vi "ELVIS III v1.0 Reset Encoder.vi"(8 "error in (no error)":errorcluster, 10 "Channel":T1, 11 "myRIO Ref In":T2) -> (0 "error out":errorcluster, 3 "myRIO Ref Out":T2)   [LabVIEW 2021]
uses:
  <vilib>/myRIO/Common/Instrument Driver Framework/Utilities/typedefs/myRIO v1.0 Reference.ctl
  <vilib>/myRIO/Common/Instrument Driver Framework/Utilities/typedefs/Generic FPGA Reference.ctl
  <vilib>/myRIO/Common/Instrument Driver Framework/myRIO v1.0/Encoder/typedefs/Encoder Channels Enum.ctl
  <vilib>/myRIO/Common/Instrument Driver Framework/ELVIS III v1.0/Encoder/typedefs/ELVIS III Encoder Channels FPGA Reference.ctl
  <vilib>/rvi/errors/niLvFpgaAdjustHostInterfaceError.vi
  <vilib>/rvi/interface/nirviReadWriteControl/nirviReadWriteControl.xnode
  <vilib>/rvi/interface/Simulation/niFpgaSimulationCallBeginRW.vi
  NiFpgaLv.dll
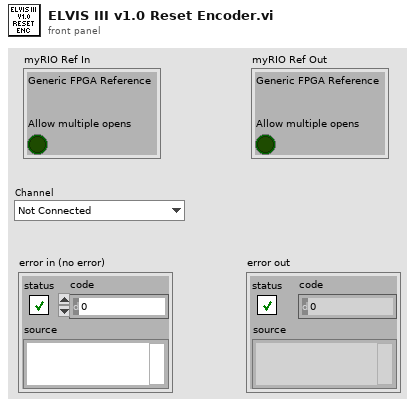
[diagram p1: front panel]
types:
  T1 = typedef "Encoder Channels Enum.ctl" = enum16{"Not Connected", "C/ENC0", "C/ENC1", "A/ENC", "A/ENC0", "A/ENC1", "A/ENC2", "A/ENC3", "A/ENC4", "A/ENC5", "A/ENC6", "A/ENC7", "A/ENC8", "A/ENC9", "B/ENC", "B/ENC0", "B/ENC1", "B/ENC2", "B/ENC3", "B/ENC4", "B/ENC5", "B/ENC6", "B/ENC7", "B/ENC8", "B/ENC9", "DIO/ENC0", "DIO/ENC1", "DIO/ENC2", "DIO/ENC3", "DIO/ENC4"}
  T2 = typedef "myRIO v1.0 Reference.ctl" = cluster{"Generic FPGA Reference":T3, "Allow multiple opens":bool}
  T3 = typedef "Generic FPGA Reference.ctl" = refnum<k20>
  T4 = typedef "ELVIS III Encoder Channels FPGA Reference.ctl" = refnum<k20>
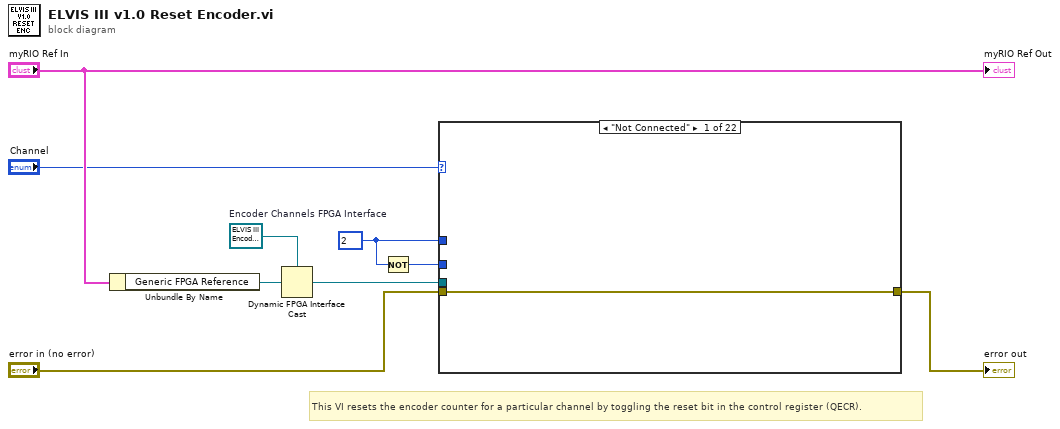
[diagram p0: block diagram]
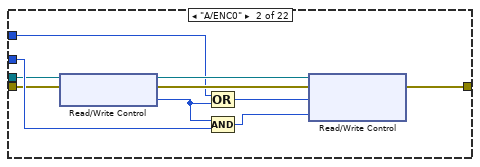
[diagram p2: hidden frame]
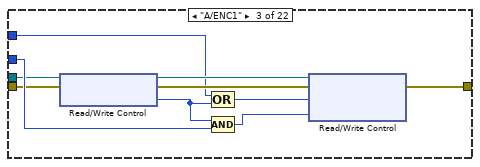
[diagram p3: hidden frame]
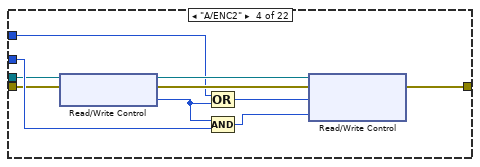
[diagram p4: hidden frame]
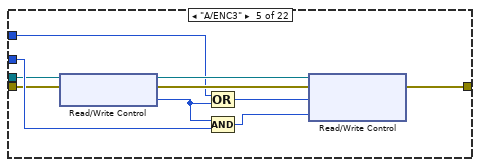
[diagram p5: hidden frame]
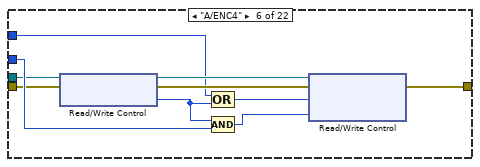
[diagram p6: hidden frame]
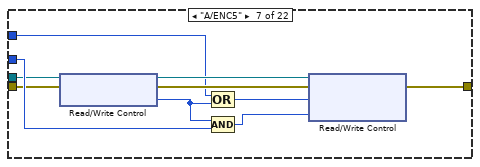
[diagram p7: hidden frame]
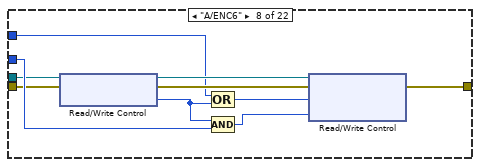
[diagram p8: hidden frame]
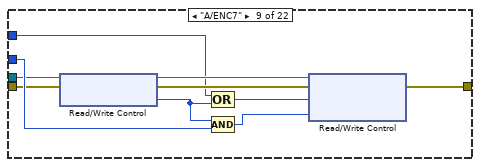
[diagram p9: hidden frame]
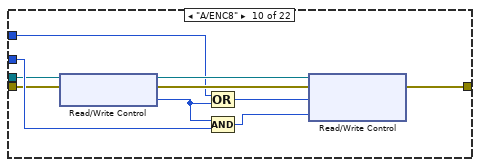
[diagram p10: hidden frame]
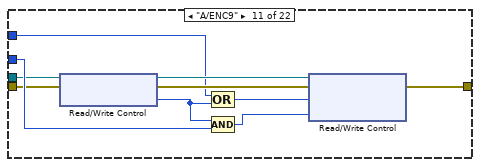
[diagram p11: hidden frame]
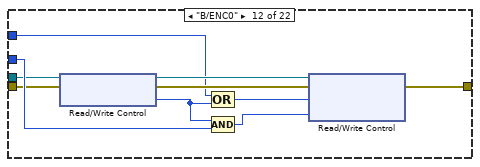
[diagram p12: hidden frame]
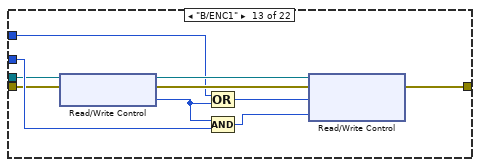
[diagram p13: hidden frame]
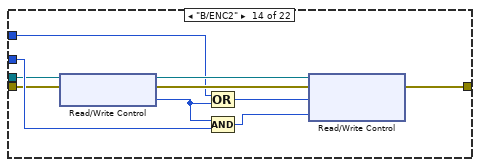
[diagram p14: hidden frame]
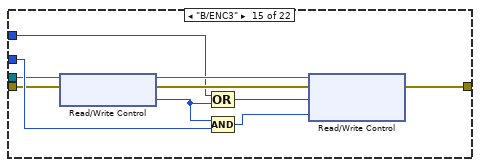
[diagram p15: hidden frame]
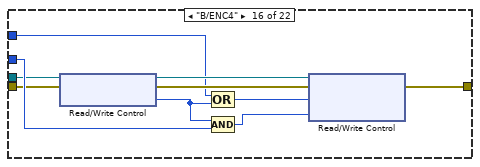
[diagram p16: hidden frame]
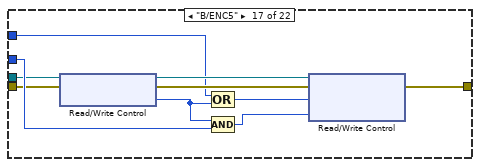
[diagram p17: hidden frame]
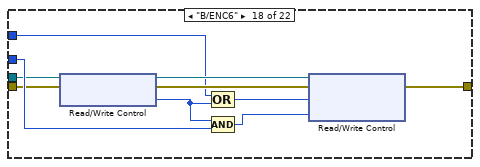
[diagram p18: hidden frame]
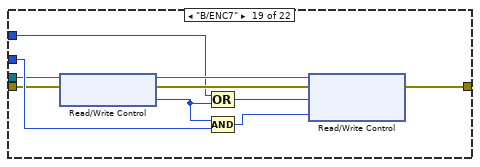
[diagram p19: hidden frame]
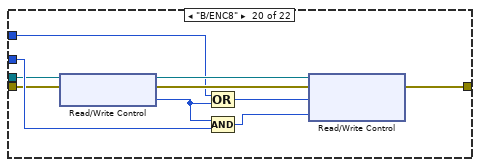
[diagram p20: hidden frame]
diagram:
  w4 = u8 2
  w9 = T4 refnum  # Encoder Channels FPGA Interface
  # "This VI resets the encoder counter for a particular channel by toggling the reset bit in the control register (QECR)."
  n1 = Unbundle By Name("myRIO Ref In") -> ("Generic FPGA Reference"=w8:T3)
  n2 = Dynamic FPGA Interface Cast(Session In=w9, Type=w8) -> (Session Out=w2:T4)
  n3 = Not(x=w4) -> (.not. x?=w3:u8)
  n4 = case shown="\"Not Connected\"" "Channel" {
    tunnel: "error in (no error)" -> [w10 w13 w23 w33 w43 w53 w63 w73 w83 w93 w103 w113 w123 w133 w143 w153 w163 w173 w183 w193 w203 w212]
    tunnel: [w10 w12 w22 w32 w42 w52 w62 w72 w82 w92 w102 w112 w122 w132 w142 w152 w162 w172 w182 w192 w202 w211] -> w5
    tunnel: w4 -> [_ w15 w25 w35 w45 w55 w65 w75 w85 w95 w105 w115 w125 w135 w145 w155 w165 w175 w185 w195 w205 _]
    tunnel: w3 -> [_ w14 w24 w34 w44 w54 w64 w74 w84 w94 w104 w114 w124 w134 w144 w154 w164 w174 w184 w194 w204 _]
    tunnel: w2 -> [_ w11 w21 w31 w41 w51 w61 w71 w81 w91 w101 w111 w121 w131 w141 w151 w161 w171 w181 w191 w201 _]
    frame "Not Connected" {
    }
    frame "A/ENC0" {
      n5 = xnode "Read/Write Control"("FPGA VI Reference In"=w11, "error in"=w13) -> ("FPGA VI Reference Out"=w19:T4, "error out"=w18:errorcluster, "ENC.A_0.CNFG"=w20:u8)
      n6 = Compound Arithmetic op=OR(w15, w20) -> (w17:u8)
      n7 = Compound Arithmetic op=AND(w20, w14) -> (w16:u8)
      n8 = xnode "Read/Write Control"("FPGA VI Reference In"=w19, "error in"=w18, "ENC.A_0.CNFG"=w17, "ENC.A_0.CNFG"=w16) -> ("error out"=w12:errorcluster)  [unwired: 1 out]
    }
    frame "A/ENC1" {
      n9 = xnode "Read/Write Control"("FPGA VI Reference In"=w21, "error in"=w23) -> ("FPGA VI Reference Out"=w29:T4, "error out"=w28:errorcluster, "ENC.A_1.CNFG"=w30:u8)
      n10 = Compound Arithmetic op=OR(w25, w30) -> (w27:u8)
      n11 = Compound Arithmetic op=AND(w30, w24) -> (w26:u8)
      n12 = xnode "Read/Write Control"("FPGA VI Reference In"=w29, "error in"=w28, "ENC.A_1.CNFG"=w27, "ENC.A_1.CNFG"=w26) -> ("error out"=w22:errorcluster)  [unwired: 1 out]
    }
    frame "A/ENC2" {
      n13 = xnode "Read/Write Control"("FPGA VI Reference In"=w31, "error in"=w33) -> ("FPGA VI Reference Out"=w39:T4, "error out"=w38:errorcluster, "ENC.A_2.CNFG"=w40:u8)
      n14 = Compound Arithmetic op=OR(w35, w40) -> (w37:u8)
      n15 = Compound Arithmetic op=AND(w40, w34) -> (w36:u8)
      n16 = xnode "Read/Write Control"("FPGA VI Reference In"=w39, "error in"=w38, "ENC.A_2.CNFG"=w37, "ENC.A_2.CNFG"=w36) -> ("error out"=w32:errorcluster)  [unwired: 1 out]
    }
    frame "A/ENC3" {
      n17 = xnode "Read/Write Control"("FPGA VI Reference In"=w41, "error in"=w43) -> ("FPGA VI Reference Out"=w49:T4, "error out"=w48:errorcluster, "ENC.A_3.CNFG"=w50:u8)
      n18 = Compound Arithmetic op=OR(w45, w50) -> (w47:u8)
      n19 = Compound Arithmetic op=AND(w50, w44) -> (w46:u8)
      n20 = xnode "Read/Write Control"("FPGA VI Reference In"=w49, "error in"=w48, "ENC.A_3.CNFG"=w47, "ENC.A_3.CNFG"=w46) -> ("error out"=w42:errorcluster)  [unwired: 1 out]
    }
    frame "A/ENC4" {
      n21 = xnode "Read/Write Control"("FPGA VI Reference In"=w51, "error in"=w53) -> ("FPGA VI Reference Out"=w59:T4, "error out"=w58:errorcluster, "ENC.A_4.CNFG"=w60:u8)
      n22 = Compound Arithmetic op=OR(w55, w60) -> (w57:u8)
      n23 = Compound Arithmetic op=AND(w60, w54) -> (w56:u8)
      n24 = xnode "Read/Write Control"("FPGA VI Reference In"=w59, "error in"=w58, "ENC.A_4.CNFG"=w57, "ENC.A_4.CNFG"=w56) -> ("error out"=w52:errorcluster)  [unwired: 1 out]
    }
    frame "A/ENC5" {
      n25 = xnode "Read/Write Control"("FPGA VI Reference In"=w61, "error in"=w63) -> ("FPGA VI Reference Out"=w69:T4, "error out"=w68:errorcluster, "ENC.A_5.CNFG"=w70:u8)
      n26 = Compound Arithmetic op=OR(w65, w70) -> (w67:u8)
      n27 = Compound Arithmetic op=AND(w70, w64) -> (w66:u8)
      n28 = xnode "Read/Write Control"("FPGA VI Reference In"=w69, "error in"=w68, "ENC.A_5.CNFG"=w67, "ENC.A_5.CNFG"=w66) -> ("error out"=w62:errorcluster)  [unwired: 1 out]
    }
    frame "A/ENC6" {
      n29 = xnode "Read/Write Control"("FPGA VI Reference In"=w71, "error in"=w73) -> ("FPGA VI Reference Out"=w79:T4, "error out"=w78:errorcluster, "ENC.A_6.CNFG"=w80:u8)
      n30 = Compound Arithmetic op=OR(w75, w80) -> (w77:u8)
      n31 = Compound Arithmetic op=AND(w80, w74) -> (w76:u8)
      n32 = xnode "Read/Write Control"("FPGA VI Reference In"=w79, "error in"=w78, "ENC.A_6.CNFG"=w77, "ENC.A_6.CNFG"=w76) -> ("error out"=w72:errorcluster)  [unwired: 1 out]
    }
    frame "A/ENC7" {
      n33 = xnode "Read/Write Control"("FPGA VI Reference In"=w81, "error in"=w83) -> ("FPGA VI Reference Out"=w89:T4, "error out"=w88:errorcluster, "ENC.A_7.CNFG"=w90:u8)
      n34 = Compound Arithmetic op=OR(w85, w90) -> (w87:u8)
      n35 = Compound Arithmetic op=AND(w90, w84) -> (w86:u8)
      n36 = xnode "Read/Write Control"("FPGA VI Reference In"=w89, "error in"=w88, "ENC.A_7.CNFG"=w87, "ENC.A_7.CNFG"=w86) -> ("error out"=w82:errorcluster)  [unwired: 1 out]
    }
    frame "A/ENC8" {
      n37 = xnode "Read/Write Control"("FPGA VI Reference In"=w91, "error in"=w93) -> ("FPGA VI Reference Out"=w99:T4, "error out"=w98:errorcluster, "ENC.A_8.CNFG"=w100:u8)
      n38 = Compound Arithmetic op=OR(w95, w100) -> (w97:u8)
      n39 = Compound Arithmetic op=AND(w100, w94) -> (w96:u8)
      n40 = xnode "Read/Write Control"("FPGA VI Reference In"=w99, "error in"=w98, "ENC.A_8.CNFG"=w97, "ENC.A_8.CNFG"=w96) -> ("error out"=w92:errorcluster)  [unwired: 1 out]
    }
    frame "A/ENC9" {
      n41 = xnode "Read/Write Control"("FPGA VI Reference In"=w101, "error in"=w103) -> ("FPGA VI Reference Out"=w109:T4, "error out"=w108:errorcluster, "ENC.A_9.CNFG"=w110:u8)
      n42 = Compound Arithmetic op=OR(w105, w110) -> (w107:u8)
      n43 = Compound Arithmetic op=AND(w110, w104) -> (w106:u8)
      n44 = xnode "Read/Write Control"("FPGA VI Reference In"=w109, "error in"=w108, "ENC.A_9.CNFG"=w107, "ENC.A_9.CNFG"=w106) -> ("error out"=w102:errorcluster)  [unwired: 1 out]
    }
    frame "B/ENC0" {
      n45 = xnode "Read/Write Control"("FPGA VI Reference In"=w111, "error in"=w113) -> ("FPGA VI Reference Out"=w119:T4, "error out"=w118:errorcluster, "ENC.B_0.CNFG"=w120:u8)
      n46 = Compound Arithmetic op=OR(w115, w120) -> (w117:u8)
      n47 = Compound Arithmetic op=AND(w120, w114) -> (w116:u8)
      n48 = xnode "Read/Write Control"("FPGA VI Reference In"=w119, "error in"=w118, "ENC.B_0.CNFG"=w117, "ENC.B_0.CNFG"=w116) -> ("error out"=w112:errorcluster)  [unwired: 1 out]
    }
    frame "B/ENC1" {
      n49 = xnode "Read/Write Control"("FPGA VI Reference In"=w121, "error in"=w123) -> ("FPGA VI Reference Out"=w129:T4, "error out"=w128:errorcluster, "ENC.B_1.CNFG"=w130:u8)
      n50 = Compound Arithmetic op=OR(w125, w130) -> (w127:u8)
      n51 = Compound Arithmetic op=AND(w130, w124) -> (w126:u8)
      n52 = xnode "Read/Write Control"("FPGA VI Reference In"=w129, "error in"=w128, "ENC.B_1.CNFG"=w127, "ENC.B_1.CNFG"=w126) -> ("error out"=w122:errorcluster)  [unwired: 1 out]
    }
    frame "B/ENC2" {
      n53 = xnode "Read/Write Control"("FPGA VI Reference In"=w131, "error in"=w133) -> ("FPGA VI Reference Out"=w139:T4, "error out"=w138:errorcluster, "ENC.B_2.CNFG"=w140:u8)
      n54 = Compound Arithmetic op=OR(w135, w140) -> (w137:u8)
      n55 = Compound Arithmetic op=AND(w140, w134) -> (w136:u8)
      n56 = xnode "Read/Write Control"("FPGA VI Reference In"=w139, "error in"=w138, "ENC.B_2.CNFG"=w137, "ENC.B_2.CNFG"=w136) -> ("error out"=w132:errorcluster)  [unwired: 1 out]
    }
    frame "B/ENC3" {
      n57 = xnode "Read/Write Control"("FPGA VI Reference In"=w141, "error in"=w143) -> ("FPGA VI Reference Out"=w149:T4, "error out"=w148:errorcluster, "ENC.B_3.CNFG"=w150:u8)
      n58 = Compound Arithmetic op=OR(w145, w150) -> (w147:u8)
      n59 = Compound Arithmetic op=AND(w150, w144) -> (w146:u8)
      n60 = xnode "Read/Write Control"("FPGA VI Reference In"=w149, "error in"=w148, "ENC.B_3.CNFG"=w147, "ENC.B_3.CNFG"=w146) -> ("error out"=w142:errorcluster)  [unwired: 1 out]
    }
    frame "B/ENC4" {
      n61 = xnode "Read/Write Control"("FPGA VI Reference In"=w151, "error in"=w153) -> ("FPGA VI Reference Out"=w159:T4, "error out"=w158:errorcluster, "ENC.B_4.CNFG"=w160:u8)
      n62 = Compound Arithmetic op=OR(w155, w160) -> (w157:u8)
      n63 = Compound Arithmetic op=AND(w160, w154) -> (w156:u8)
      n64 = xnode "Read/Write Control"("FPGA VI Reference In"=w159, "error in"=w158, "ENC.B_4.CNFG"=w157, "ENC.B_4.CNFG"=w156) -> ("error out"=w152:errorcluster)  [unwired: 1 out]
    }
    frame "B/ENC5" {
      n65 = xnode "Read/Write Control"("FPGA VI Reference In"=w161, "error in"=w163) -> ("FPGA VI Reference Out"=w169:T4, "error out"=w168:errorcluster, "ENC.B_5.CNFG"=w170:u8)
      n66 = Compound Arithmetic op=OR(w165, w170) -> (w167:u8)
      n67 = Compound Arithmetic op=AND(w170, w164) -> (w166:u8)
      n68 = xnode "Read/Write Control"("FPGA VI Reference In"=w169, "error in"=w168, "ENC.B_5.CNFG"=w167, "ENC.B_5.CNFG"=w166) -> ("error out"=w162:errorcluster)  [unwired: 1 out]
    }
    frame "B/ENC6" {
      n69 = xnode "Read/Write Control"("FPGA VI Reference In"=w171, "error in"=w173) -> ("FPGA VI Reference Out"=w179:T4, "error out"=w178:errorcluster, "ENC.B_6.CNFG"=w180:u8)
      n70 = Compound Arithmetic op=OR(w175, w180) -> (w177:u8)
      n71 = Compound Arithmetic op=AND(w180, w174) -> (w176:u8)
      n72 = xnode "Read/Write Control"("FPGA VI Reference In"=w179, "error in"=w178, "ENC.B_6.CNFG"=w177, "ENC.B_6.CNFG"=w176) -> ("error out"=w172:errorcluster)  [unwired: 1 out]
    }
    frame "B/ENC7" {
      n73 = xnode "Read/Write Control"("FPGA VI Reference In"=w181, "error in"=w183) -> ("FPGA VI Reference Out"=w189:T4, "error out"=w188:errorcluster, "ENC.B_7.CNFG"=w190:u8)
      n74 = Compound Arithmetic op=OR(w185, w190) -> (w187:u8)
      n75 = Compound Arithmetic op=AND(w190, w184) -> (w186:u8)
      n76 = xnode "Read/Write Control"("FPGA VI Reference In"=w189, "error in"=w188, "ENC.B_7.CNFG"=w187, "ENC.B_7.CNFG"=w186) -> ("error out"=w182:errorcluster)  [unwired: 1 out]
    }
    frame "B/ENC8" {
      n77 = xnode "Read/Write Control"("FPGA VI Reference In"=w191, "error in"=w193) -> ("FPGA VI Reference Out"=w199:T4, "error out"=w198:errorcluster, "ENC.B_8.CNFG"=w200:u8)
      n78 = Compound Arithmetic op=OR(w195, w200) -> (w197:u8)
      n79 = Compound Arithmetic op=AND(w200, w194) -> (w196:u8)
      n80 = xnode "Read/Write Control"("FPGA VI Reference In"=w199, "error in"=w198, "ENC.B_8.CNFG"=w197, "ENC.B_8.CNFG"=w196) -> ("error out"=w192:errorcluster)  [unwired: 1 out]
    }
    frame "B/ENC9" {
      n81 = xnode "Read/Write Control"("FPGA VI Reference In"=w201, "error in"=w203) -> ("FPGA VI Reference Out"=w209:T4, "error out"=w208:errorcluster, "ENC.B_9.CNFG"=w210:u8)
      n82 = Compound Arithmetic op=OR(w205, w210) -> (w207:u8)
      n83 = Compound Arithmetic op=AND(w210, w204) -> (w206:u8)
      n84 = xnode "Read/Write Control"("FPGA VI Reference In"=w209, "error in"=w208, "ENC.B_9.CNFG"=w207, "ENC.B_9.CNFG"=w206) -> ("error out"=w202:errorcluster)  [unwired: 1 out]
    }
    frame Default {
      # "The channel requested is not supported. This happens when the channel name is valid (a valid channel enum) but there it is not handled in the case structure."
      n85 = call <vilib>:"Error Cluster From Error Code.vi"("error in (no error)"=w212, "error code (0)"=-363003) -> ("error out"=w211:errorcluster)  [unwired: 7 in]
    }
  }
  "error out" <- w5
  "myRIO Ref Out" <- "myRIO Ref In"
